vi "Page_Hardware_Read.vi"(6 "ctlReferences":T1, 8 "error in (no error)":errorcluster, 11 "Class in":refnum<class "IB_MSI.lvclass">) -> (0 "error out":errorcluster, 3 "Class out":refnum<class "IB_MSI.lvclass">)   [LabVIEW 2020, in "IB_MSI.lvclass"]
uses:
  <vilib>/AppBuilder/IB_Classes/MSI/IB_MSI.lvclass
  <resource>/Framework/Providers/Builds/Installer/Pages/controls/IB_UI_Page_Hardware_References.ctl
  <vilib>/AppBuilder/IB_Classes/MSI/IB_MSI.lvclass/IB_MSI.ctl
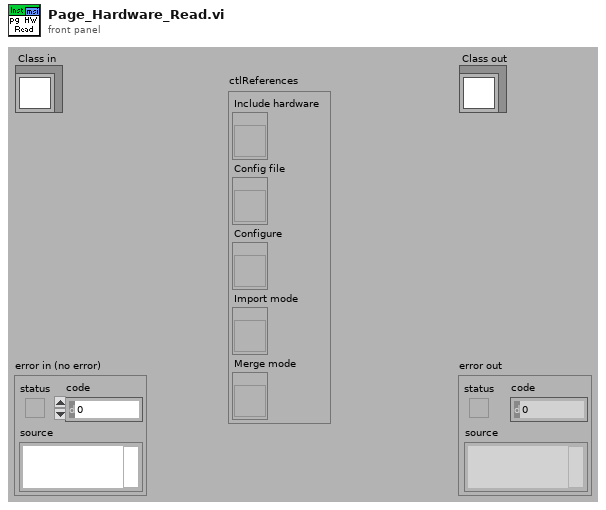
[diagram p1: front panel]
types:
  T1 = typedef "IB_UI_Page_Hardware_References.ctl" = cluster{"Include hardware":refnum<vi>, "Config file":refnum<vi>, "Configure":refnum<vi>, "Import mode":refnum<vi>, "Merge mode":refnum<vi>}
  T2 = typedef "CDK_sTypeDef_HWImportOption.ctl" = enum16{"<none>", "Merge", "Replace", "Dialog"}
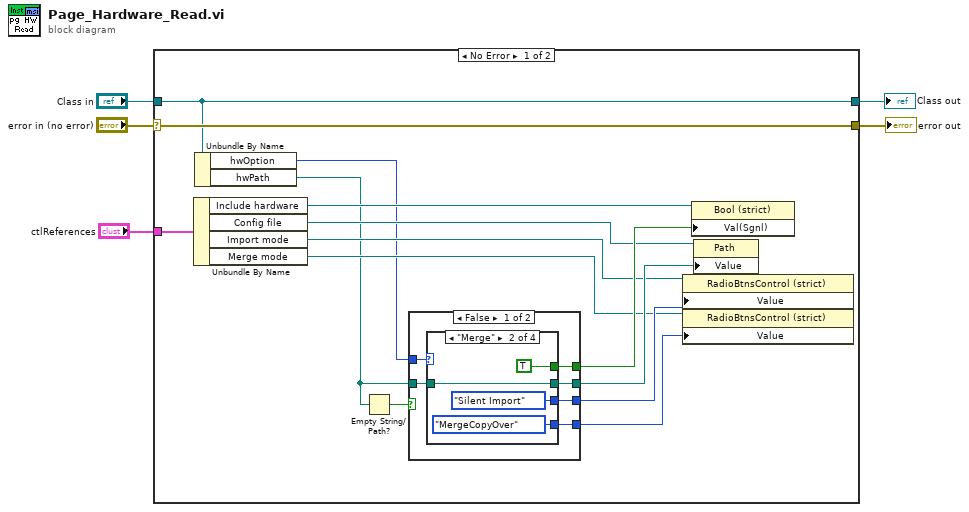
[diagram p0: block diagram]
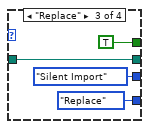
[diagram p3: hidden frame]
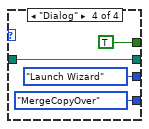
[diagram p4: hidden frame]
diagram:
  n1 = case shown="No Error" "error in (no error)" {
    selector: "error in (no error)" -> [w19 w39]
    tunnel: [w19 w39] -> w4
    tunnel: [w9 w38] -> w2
    tunnel: "Class in" -> [w9 w38]
    tunnel: "ctlReferences" -> [w8 _]
    frame No Error {
      n2 = Unbundle By Name(w8) -> ("Include hardware"=w13:refnum<vi>, "Config file"=w12:refnum<vi>, "Import mode"=w11:refnum<vi>, "Merge mode"=w10:refnum<vi>)
      n3 = Unbundle By Name(w9) -> ("hwOption"=w7:T2, "hwPath"=w6:path)
      n4 = Empty String/Path?(string/path=w6) -> (empty?=w16:bool)
      n5 = case shown="False" w16 {
        tunnel: w7 -> [w25 _]
        tunnel: [w24 _] -> w18
        tunnel: [w23 _] -> w17
        tunnel: w6 -> [w22 _]
        tunnel: [w21 _] -> w15
        tunnel: [w20 _] -> w14
        frame False {
          n6 = case shown="\"Merge\"" w25 {
            tunnel: w22 -> [_ w29 w33 w37]
            tunnel: [_ w29 w33 w37] -> w24
            tunnel: [_ TRUE TRUE TRUE] -> w23
            tunnel: [_ enum32{"Launch Wizard", "Silent Import"}."Silent Import" ("Value") enum32{"Launch Wizard", "Silent Import"}."Silent Import" ("Value") enum32{"Launch Wizard", "Silent Import"}."Launch Wizard" ("Value")] -> w21
            tunnel: [_ enum32{"MergeCopyOver", "Replace"}."MergeCopyOver" ("Value") enum32{"MergeCopyOver", "Replace"}."Replace" ("Value") enum32{"MergeCopyOver", "Replace"}."MergeCopyOver" ("Value")] -> w20
            frame "<none>" {
            }
            frame "Merge" {
            }
            frame "Replace" {
            }
            frame "Dialog" {
            }
          }
        }
        frame True {
        }
      }
      n7 = property class="RadioBtnsControl (strict)"(reference=w11, "Value"=w15) -> ()  [unwired: 1 in, 2 out]
      n8 = property class="RadioBtnsControl (strict)"(reference=w10, "Value"=w14) -> ()  [unwired: 1 in, 2 out]
      n9 = property class="Bool (strict)"(reference=w13, "Val(Sgnl)"=w17) -> ()  [unwired: 1 in, 2 out]
      n10 = property class="Path"(reference=w12, "Value"=w18) -> ()  [unwired: 1 in, 2 out]
    }
    frame Error {
    }
  }
  "error out" <- w4
  "Class out" <- w2
